vi "gugudan Client.vi"() -> ()   [LabVIEW 2014]
uses:
  <vilib>/Utility/sysdir.llb/System Directory Type.ctl
  <vilib>/FTP/NI_FTP.lvlib
panel:
  out "ip address 3":string=" ip address\r\n   서브넷 마스크 . . . . . . . : 255.255.255.0\r\n   기본 게이트웨이 . . . . . . : 192.168.0.1\r\n\r\n터널 어댑터 isatap.{E2E91750-802C-47E4-94E7-F6C5BD44A78B}:\r\n\r\n   미디어 상태 . . . . . . . . : 미디어 연결 끊김\r\n   연결별 DNS 접미사. . . . : \r\n\r\n터널 어댑터 로컬 영역 연결* 2:\r\n\r\n   연결별 DNS 접미사. . . . : \r\n   IPv6 주소 . . . . . . . . . : 2001:0:682f:9980:3c40:17a9:3f57:fff6\r\n   링크-로컬 IPv6 주소 . . . . : fe80::3c40:17a9:3f57:fff6%12\r\n   기본 게이트웨이 . . . . . . : ::\r\n"
  out "email 2":string
  out "ip address":string=" ip address\r\n   서브넷 마스크 . . . . . . . : 255.255.255.0\r\n   기본 게이트웨이 . . . . . . : 192.168.0.1\r\n\r\n터널 어댑터 isatap.{E2E91750-802C-47E4-94E7-F6C5BD44A78B}:\r\n\r\n   미디어 상태 . . . . . . . . : 미디어 연결 끊김\r\n   연결별 DNS 접미사. . . . : \r\n\r\n터널 어댑터 로컬 영역 연결* 2:\r\n\r\n   연결별 DNS 접미사. . . . : \r\n   IPv6 주소 . . . . . . . . . : 2001:0:682f:9980:3c40:17a9:3f57:fff6\r\n   링크-로컬 IPv6 주소 . . . . : fe80::3c40:17a9:3f57:fff6%12\r\n   기본 게이트웨이 . . . . . . : ::\r\n"
  in  "제한해제":bool
  out "TIME":string="현재날자,시간"
  out "배열":string[][](array[string])
  out "email":string
  out "abs(x)":i32
  out "문자열":string
  out "스페이스바3 2":string
  out "W 2":string
  out "W":string
  out "1":string
  out "2":string
  out "3":string
  out "스페이스바3":string
  out "key의숫자값":i16[](array[numeric])
  # "서비스를 이용해 주셔 감사합니다."
  # "서비스 종료를 위해서는 관리자 암호를 입력 해야 종료가 가능합니다."
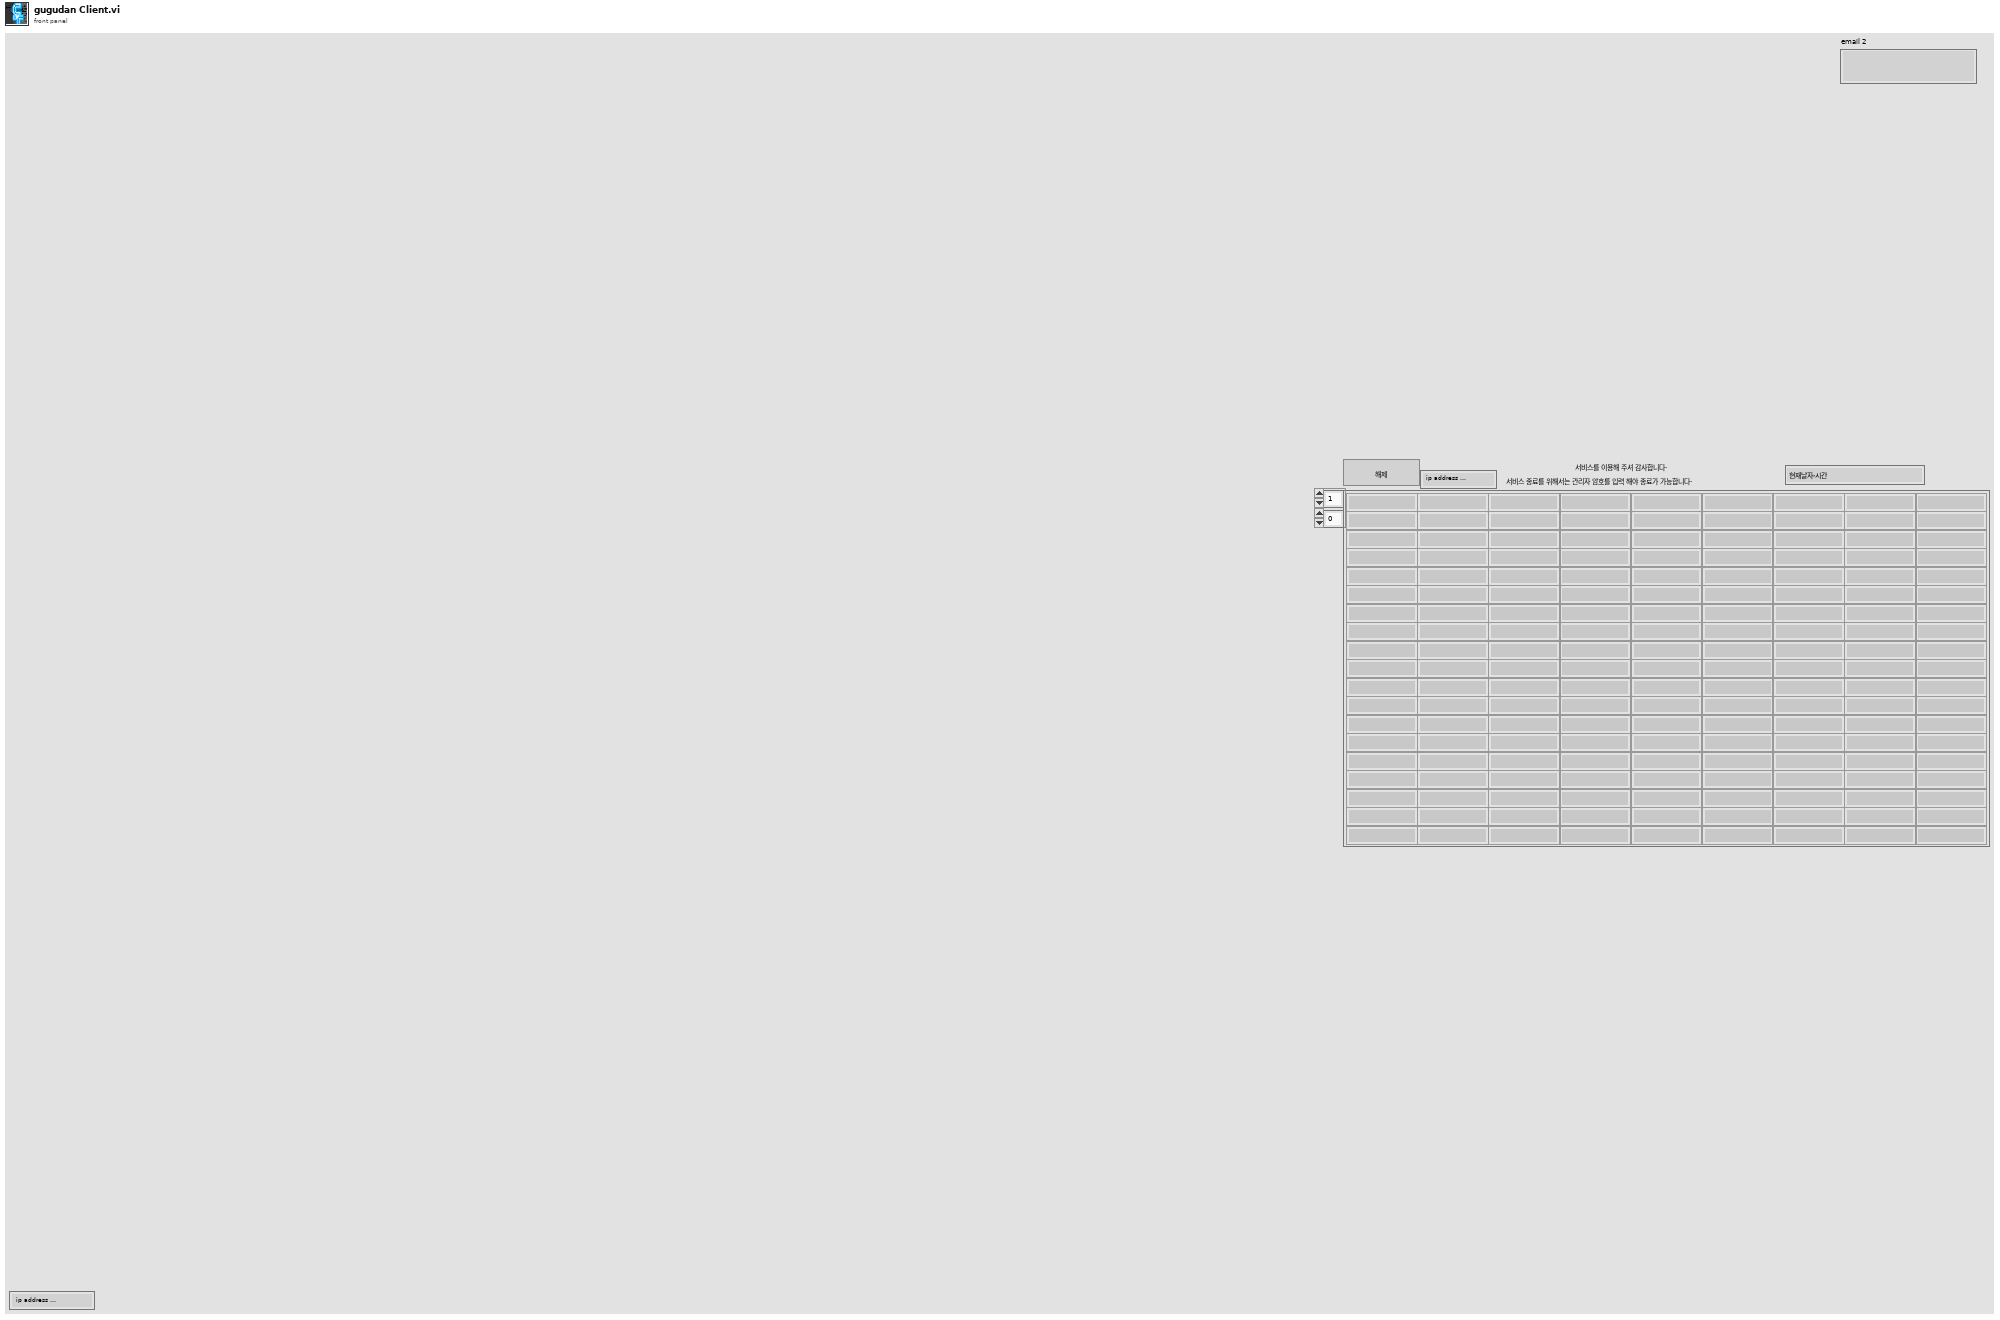
[diagram p1: front panel]
types:
  T1 = enum16{"open", "replace", "create", "open or create", "replace or create", "replace or create with confirmation"}
  T2 = typedef "NI_FTP.lvlib/FTP Session.ctl" = refnum<k5>
  T3 = typedef "System Directory Type.ctl" = i32
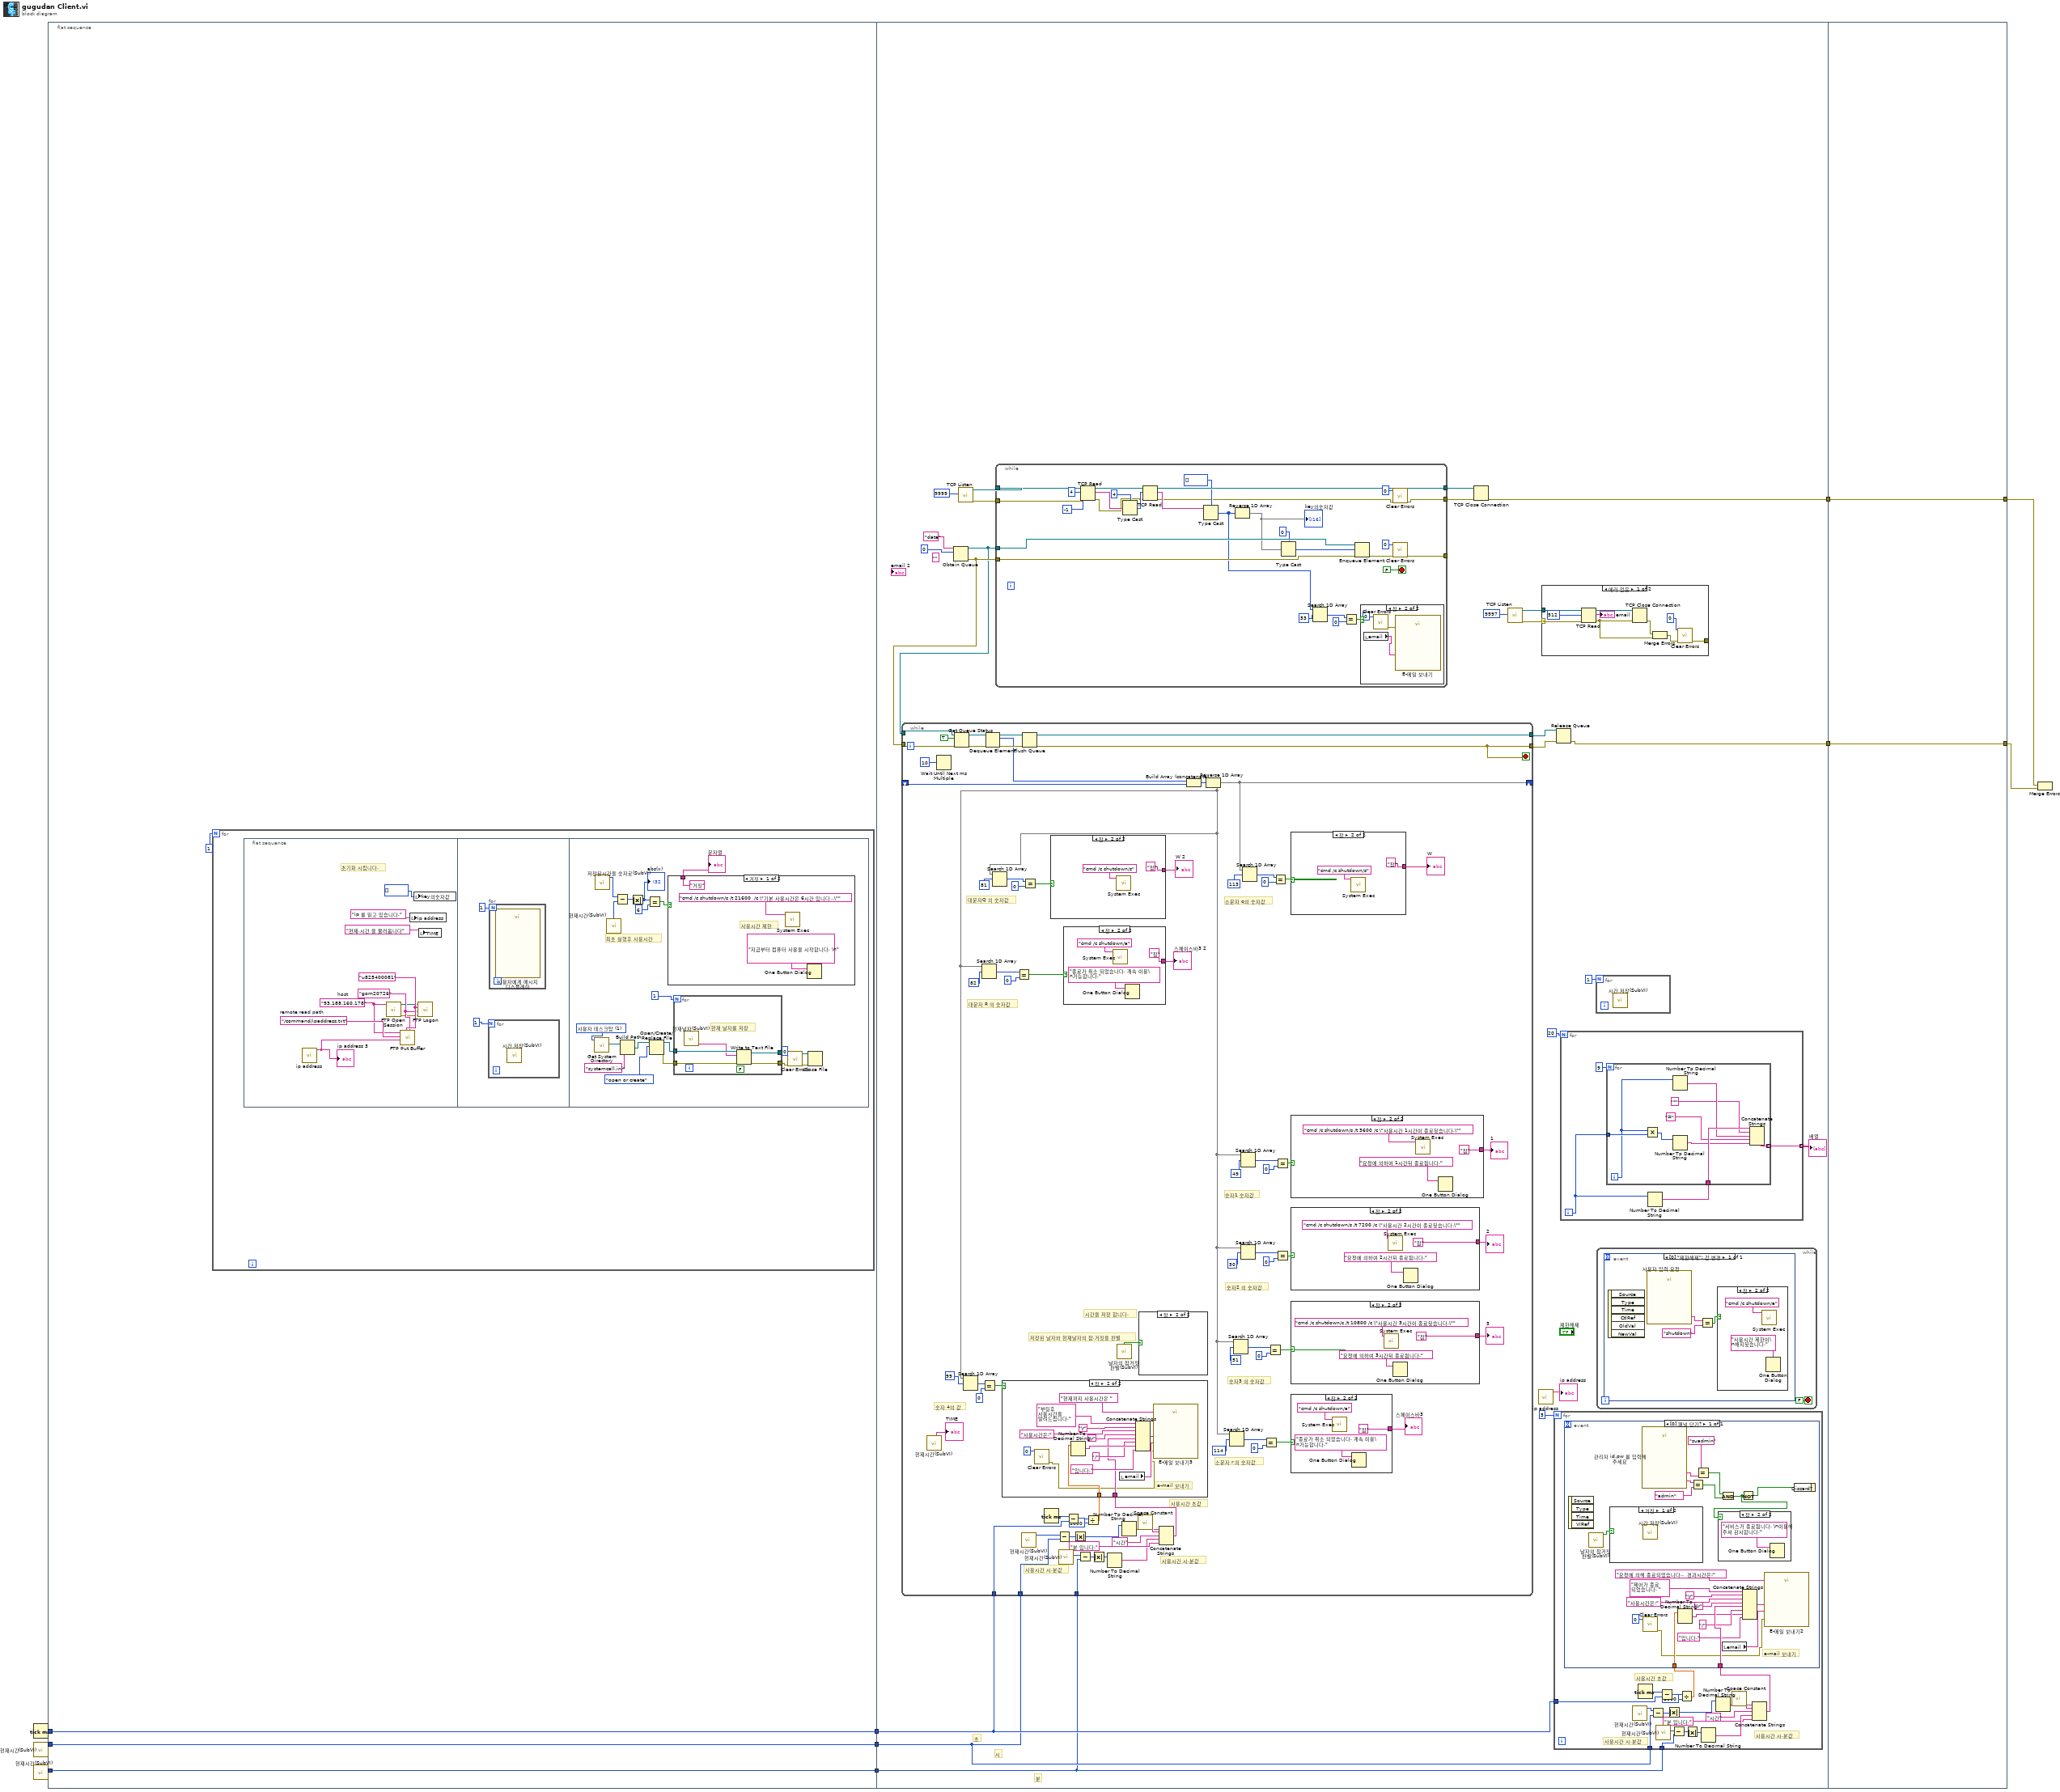
[diagram p0: block diagram]
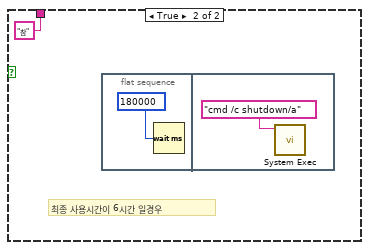
[diagram p2: hidden frame]
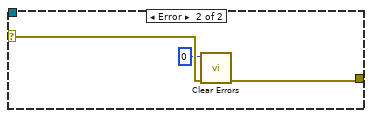
[diagram p4: hidden frame]
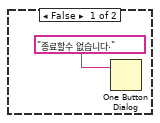
[diagram p6: hidden frame]
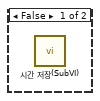
[diagram p8: hidden frame]
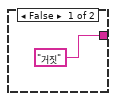
[diagram p9: hidden frame]
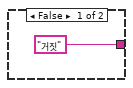
[diagram p10: hidden frame]
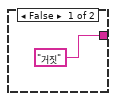
[diagram p11: hidden frame]
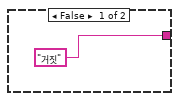
[diagram p12: hidden frame]
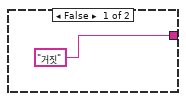
[diagram p13: hidden frame]
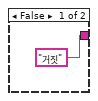
[diagram p14: hidden frame]
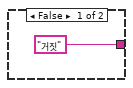
[diagram p15: hidden frame]
diagram:
  n1 = Tick Count (ms)() -> (millisecond timer value=w6:u32)
  n2 = call "현재시간(SubVI).vi"() -> ("시"=w5:i32)  [unwired: 3 in, 8 out]
  n3 = call "현재시간(SubVI).vi"() -> ("분"=w4:i32)  [unwired: 3 in, 8 out]
  n4 = flat-sequence {
    tunnel: [w13] -> w7
    tunnel: w6 -> [w13]
    tunnel: w5 -> [w12]
    tunnel: w4 -> [w11]
    tunnel: [w12] -> w3
    tunnel: [w11] -> w2
    tunnel: [w71] -> w10
    tunnel: [w70] -> w9
    tunnel: w7 -> [w66]
    tunnel: w3 -> [w65]
    tunnel: w2 -> [w64]
    tunnel: w10 -> [w304]
    tunnel: w9 -> [w303]
    tunnel: [w304] -> w8
    tunnel: [w303] -> w1
    frame #0 {
      n5 = for {
        N: 1 -> [_]
        n6 = flat-sequence {
          frame #0 {
            w17 = "gom20726"
            w20 = "u825400081"
            w19 = "/command/ipaddress.txt"  # remote read path
            w18 = "93.188.160.178"  # host
            # "초기화 시킵니다."
            n7 = call "ip address.vi"() -> ("ip address"=w21:string)  [unwired: 11 in]
            "ip address 3" <- w21
            n8 = call <vilib>:"FTP Open Session.vi"("address"=w18) -> ("error out"=w16:errorcluster, "ftp session"=w15:T2)  [unwired: 7 in, 2 out]
            n9 = call <vilib>:"FTP Put Buffer.vi"("password"=w17, "user"=w20, "data"=w21, "remote path"=w19, "host"=w18) -> ()  [unwired: 5 in, 2 out]
            n10 = local write "ip address"("ip 를 읽고 있습니다.") -> ()
            n11 = local write "key의숫자값"(i16[] []) -> ()
            n12 = call <vilib>:"FTP Logon.vi"("error in (no error)"=w16, "password"=w17, "user"=w20, "ftp session"=w15) -> ()  [unwired: 4 in, 4 out]
            n13 = local write "TIME"("현재,시간 을 불러옵니다") -> ()
          }
          frame #1 {
            n14 = for {
              N: 1 -> [_]
              n15 = call "시간 저장(SubVI).vi"() -> ()  [unwired: 12 in]
            }
            n16 = for {
              N: 1 -> [_]
              n17 = call "사용자에게 메시지 디스플레이"() -> ()  [unwired: 10 in, 2 out]
            }
          }
          frame #2 {
            w29 = T3 1 items=["사용자 홈"=0, "사용자 데스크탑"=1, "사용자 문서"=2, "사용자 어플리케이션 데이터"=3, "사용자 환경"=4, "사용자 임시"=5, "퍼블릭 문서"=6, "퍼블릭 어플리케이션 데이터"=7, "퍼블릭 환경"=8, "퍼블릭 캐시"=13, "시스템 코어 라이브러리"=9, "시스템 설치된 라이브러리"=10, "어플리케이션 파일"=11, "부팅 볼륨 루트"=12] ("system directory type")
            # "최초 실행후 사용시간"
            n18 = call <vilib>:"Get System Directory.vi"("system directory type"=w29) -> ("system directory"=w34:path)  [unwired: 10 in]
            n19 = call "저장된시간을 숫자로(SubVI).vi"() -> ("저장된 문자를 숫자로"=w39:i32)  [unwired: 11 in]
            n20 = call "현재시간(SubVI).vi"() -> ("시"=w40:i32)  [unwired: 3 in, 8 out]
            n21 = Subtract(x=w39, y=w40) -> (x-y=w41:i32)
            n22 = Build Path(base path=w34, name or relative path="systemcall.ini" ("이름 또는 상대 경로")) -> (appended path=w32:path)
            n23 = Absolute Value(x=w41) -> (abs(x)=w43:i32)
            "abs(x)" <- w43
            n24 = Equal?(x=w43, y=6) -> (x = y?=w45:bool)
            n25 = Open/Create/Replace File(file path (use dialog)=w32, operation (0:open)=T1."open or create" ("동작(0:open)")) -> (refnum out=w30:refnum<file>, error out=w31:errorcluster)  [unwired: 4 in, 1 out]
            n26 = case shown="거짓" w45 {
              tunnel: ["거짓" "참"] -> w42
              frame False {
                # "사용시간 제한"
                n27 = call <vilib>:"System Exec.vi"("command line"="cmd /c shutdown/s /t 21600  /c \"기본 사용시간은 6시간 입니다..\"" ("standard input")) -> ()  [unwired: 7 in, 4 out]
                n28 = One Button Dialog(message="지금부터 컴퓨터 사용을 시작합니다. \n" ("메시지")) -> ()  [unwired: 1 in, 1 out]
              }
              frame True {
                # "최종 사용시간이 6시간 일경우"
                n29 = flat-sequence {
                  frame #0 {
                    n30 = Wait (ms)(milliseconds to wait=u32 180000 ("대기 시간(ms)")) -> ()  [unwired: 1 out]
                  }
                  frame #1 {
                    n31 = call <vilib>:"System Exec.vi"("command line"="cmd /c shutdown/a" ("standard input")) -> ()  [unwired: 7 in, 4 out]
                  }
                }
              }
            }
            "문자열" <- w42
            n32 = for {
              N: 1 -> [_]
              tunnel: w31 -> [w50]
              tunnel: [w49] -> w36
              tunnel: [w48] -> w35
              tunnel: w30 -> [w47]
              (unwired) FALSE
              # "현재 날자를 저장"
              n33 = call "현재날자(SubVI).vi"() -> ("월,일 을 문자열로"=w46:string)  [unwired: 5 in, 6 out]
              n34 = Write to Text File(file (use dialog)=w47, text=w46, error in=w50) -> (refnum out=w48:refnum<file>, error out=w49:errorcluster)  [unwired: 1 in, 1 out]
            }
            n35 = call <vilib>:"Clear Errors.vi"("error in (no error)"=w36, "specific error code to clear (0: all)"=0) -> ("error out"=w37:errorcluster)  [unwired: 4 in, 1 out]
            n36 = Close File(refnum=w35, error in=w37) -> ()  [unwired: 2 out]
          }
        }
      }
    }
    frame #1 {
      (unwired) ""
      # "초"
      # "분"
      # "시"
      n37 = Obtain Queue(name (unnamed)="data" ("이름(이름없음)"), element data type=i16 0) -> (queue out=w72:refnum<queue>, error out=w73:errorcluster)  [unwired: 3 in, 1 out]
      n38 = while {
        shift-right: [w158] -> _
        shift-left: _ -> [w204]
        tunnel: [w197] -> w75
        tunnel: [w196] -> w74
        tunnel: w72 -> [w203]
        tunnel: w73 -> [w202]
        tunnel: w66 -> [w163]
        tunnel: w65 -> [w162]
        tunnel: w64 -> [w161]
        stop <- w196 stop-if-true
        # "숫자 4의 값"
        # "저장된 날자와 현재날자의 참,거짓을 판별"
        # "시간을 저장 합니다."
        # "사용시간 시,분값"
        # "사용시간 시,분값"
        # "사용시간 초값"
        # "대문자 R 의 숫자값"
        # "대문자Q 의 숫자값"
        # "소문자 r 의 숫자값"
        # "숫자3 의 숫자값"
        # "소문자 q의 숫자값"
        # "숫자1 숫자값"
        # "숫자2 의 숫자값"
        n39 = call "현재시간(SubVI).vi"() -> ("날짜/시간 문자열"=→"TIME":string)  [unwired: 3 in, 8 out]
        n40 = Wait Until Next ms Multiple(millisecond multiple=u32 10) -> ()  [unwired: 1 out]
        n41 = Get Queue Status(queue=w203, return elements? (F)=TRUE ("원소 반환? (거짓)"), error in (no error)=w202) -> (queue out=w201:refnum<queue>, error out=w200:errorcluster)  [unwired: 6 out]
        n42 = Dequeue Element(queue=w201, error in (no error)=w200) -> (queue out=w198:refnum<queue>, element=w195:i16, error out=w199:errorcluster)  [unwired: 1 in, 1 out]
        n43 = call "현재시간(SubVI).vi"() -> ("시"=w165:i32)  [unwired: 3 in, 8 out]
        n44 = Flush Queue(queue=w198, error in (no error)=w199) -> (queue out=w197:refnum<queue>, error out=w196:errorcluster)  [unwired: 1 out]
        n45 = Tick Count (ms)() -> (millisecond timer value=w164:u32)
        n46 = Subtract(x=w165, y=w162) -> (x-y=w167:i32)
        n47 = call "현재시간(SubVI).vi"() -> ("분"=w166:i32)  [unwired: 3 in, 8 out]
        n48 = Subtract(x=w164, y=w163) -> (x-y=w176:u32)
        n49 = Absolute Value(x=w167) -> (abs(x)=w169:i32)
        n50 = Subtract(x=w166, y=w161) -> (x-y=w168:i32)
        n51 = Divide(x=w176, y=u32 1000) -> (x/y=w160:dbl)
        n52 = Absolute Value(x=w168) -> (abs(x)=w170:i32)
        n53 = Number To Decimal String(number=w170) -> (decimal integer string=w172:string)  [unwired: 1 in]
        n54 = call "날자의 참거짓 판별(SubVI).vi"() -> ("불리언"=w182:bool)  [unwired: 9 in, 2 out]
        n55 = Number To Decimal String(number=w169) -> (decimal integer string=w174:string)  [unwired: 1 in]
        n56 = call <vilib>:"Space Constant.vi"() -> ("String"=w175:string)
        n57 = case shown="참" w182 {
          frame False {
            n58 = call "시간 저장(SubVI).vi"() -> ()  [unwired: 12 in]
          }
          frame True {
          }
        }
        n59 = Concatenate Strings(w174, w175, "시간", w172, "분 입니다.") -> (w159:string)
        n60 = Build Array (concatenate)(w195, w204) -> (w193:i16[])
        n61 = Reverse 1D Array(array=w193) -> (reversed array=w158:i16[])
        n62 = Search 1D Array(1D array=w158, element=i16 99 ("원소")) -> (index of element=w180:i32)  [unwired: 1 in]
        n63 = Search 1D Array(1D array=w158, element=i16 82 ("원소")) -> (index of element=w185:i32)  [unwired: 1 in]
        n64 = Equal?(x=w180, y=0) -> (x = y?=w178:bool)
        n65 = Search 1D Array(1D array=w158, element=i16 81 ("원소")) -> (index of element=w190:i32)  [unwired: 1 in]
        n66 = case shown="참" w178 {
          tunnel: w160 -> [_ w235]
          tunnel: w159 -> [_ w234]
          frame False {
          }
          frame True {
            # "e-mail 보내기"
            n67 = call <vilib>:"Clear Errors.vi"("specific error code to clear (0: all)"=0) -> ("error out"=w231:errorcluster)  [unwired: 5 in, 1 out]
            n68 = Number To Decimal String(number=w235) -> (decimal integer string=w243:string)  [unwired: 1 in]
            n69 = local read "email"() -> (w233:string)
            n70 = Concatenate Strings("부팅후 사용시간을 알려드립니다." ("문자열"), "\r", "사용시간은:", "\r", w234, "/", w243, "입니다.") -> (w240:string)
            n71 = call "E-메일 보내기3"("error in"=w231, "Message"=w240, "Subject"="현재까지 사용시간은 ", "Recipients"=w233) -> ()  [unwired: 7 in, 1 out]
          }
        }
        n72 = Equal?(x=w185, y=0) -> (x = y?=w187:bool)
        n73 = Equal?(x=w190, y=0) -> (x = y?=w188:bool)
        n74 = case shown="참" w188 {
          tunnel: ["거짓" "참"] -> w192
          frame False {
          }
          frame True {
            n75 = call <vilib>:"System Exec.vi"("command line"="cmd /c shutdown/s" ("standard input")) -> ()  [unwired: 7 in, 4 out]
          }
        }
        "W 2" <- w192
        n76 = case shown="참" w187 {
          tunnel: ["거짓" "참"] -> w183
          frame False {
          }
          frame True {
            n77 = call <vilib>:"System Exec.vi"("command line"="cmd /c shutdown/a" ("standard input")) -> ()  [unwired: 7 in, 4 out]
            n78 = One Button Dialog(message="종료가 취소 되었습니다. 계속 이용\n가능합니다." ("메시지")) -> ()  [unwired: 1 in, 1 out]
          }
        }
        "스페이스바3 2" <- w183
        n79 = Search 1D Array(1D array=w158, element=i16 114 ("원소")) -> (index of element=w209:i32)  [unwired: 1 in]
        n80 = Search 1D Array(1D array=w158, element=i16 51 ("원소")) -> (index of element=w214:i32)  [unwired: 1 in]
        n81 = Search 1D Array(1D array=w158, element=i16 49 ("원소")) -> (index of element=w225:i32)  [unwired: 1 in]
        n82 = Search 1D Array(1D array=w158, element=i16 50 ("원소")) -> (index of element=w218:i32)  [unwired: 1 in]
        n83 = Search 1D Array(1D array=w158, element=i16 113 ("원소")) -> (index of element=w228:i32)  [unwired: 1 in]
        n84 = Equal?(x=w209, y=0) -> (x = y?=w211:bool)
        n85 = Equal?(x=w214, y=0) -> (x = y?=w212:bool)
        n86 = Equal?(x=w228, y=0) -> (x = y?=w226:bool)
        n87 = Equal?(x=w225, y=0) -> (x = y?=w223:bool)
        n88 = Equal?(x=w218, y=0) -> (x = y?=w220:bool)
        n89 = case shown="참" w226 {
          tunnel: ["거짓" "참"] -> w230
          frame False {
          }
          frame True {
            n90 = call <vilib>:"System Exec.vi"("command line"="cmd /c shutdown/s" ("standard input")) -> ()  [unwired: 7 in, 4 out]
          }
        }
        "W" <- w230
        n91 = case shown="참" w223 {
          tunnel: ["거짓" "참"] -> w224
          frame False {
          }
          frame True {
            n92 = call <vilib>:"System Exec.vi"("command line"="cmd /c shutdown/s /t 3600 /c \"사용시간 1시간이 종료됫습니다.\"" ("standard input")) -> ()  [unwired: 7 in, 4 out]
            n93 = One Button Dialog(message="요청에 의하여 1시간뒤 종료됩니다." ("메시지")) -> ()  [unwired: 1 in, 1 out]
          }
        }
        "1" <- w224
        n94 = case shown="참" w220 {
          tunnel: ["거짓" "참"] -> w219
          frame False {
          }
          frame True {
            n95 = call <vilib>:"System Exec.vi"("command line"="cmd /c shutdown/s /t 7200 /c \"사용시간 2시간이 종료됫습니다.\"" ("standard input")) -> ()  [unwired: 7 in, 4 out]
            n96 = One Button Dialog(message="요청에 의하여 2시간뒤 종료됩니다." ("메시지")) -> ()  [unwired: 1 in, 1 out]
          }
        }
        "2" <- w219
        n97 = case shown="참" w212 {
          tunnel: ["거짓" "참"] -> w194
          frame False {
          }
          frame True {
            n98 = call <vilib>:"System Exec.vi"("command line"="cmd /c shutdown/s /t 10800 /c \"사용시간 3시간이 종료됫습니다.\"" ("standard input")) -> ()  [unwired: 7 in, 4 out]
            n99 = One Button Dialog(message="요청에 의하여 3시간뒤 종료됩니다." ("메시지")) -> ()  [unwired: 1 in, 1 out]
          }
        }
        "3" <- w194
        n100 = case shown="참" w211 {
          tunnel: ["거짓" "참"] -> w207
          frame False {
          }
          frame True {
            n101 = call <vilib>:"System Exec.vi"("command line"="cmd /c shutdown/a" ("standard input")) -> ()  [unwired: 7 in, 4 out]
            n102 = One Button Dialog(message="종료가 취소 되었습니다. 계속 이용\n가능합니다." ("메시지")) -> ()  [unwired: 1 in, 1 out]
          }
        }
        "스페이스바3" <- w207
      }
      n103 = call <vilib>:"TCP Listen.vi"("port"=u16 9999) -> ("error out"=w68:errorcluster, "connection ID"=w78:refnum<k5>)  [unwired: 6 in, 3 out]
      n104 = while {
        tunnel: w78 -> [w271]
        tunnel: [w299] -> w79
        tunnel: w72 -> [w292]
        tunnel: w73 -> [w291]
        tunnel: [w277] -> w69
        tunnel: w68 -> [w283]
        tunnel: [w274] -> _
        stop <- FALSE stop-if-true
        n105 = TCP Read(connection ID=w271, bytes to read=4, error in (no error)=w283, 9:-1 ("타임아웃 ms (25000)")) -> (connection ID out=w295:refnum<k5>, data out=w297:string, error out=w284:errorcluster)  [unwired: 1 in]
        n106 = Type Cast(type=4 ("bytes to read"), x=w297) -> (*(type *) &x=w289:i32)
        n107 = TCP Read(connection ID=w295, bytes to read=w289, error in (no error)=w284) -> (connection ID out=w299:refnum<k5>, data out=w290:string, error out=w276:errorcluster)  [unwired: 2 in]
        n108 = Type Cast(type=i16[] [], x=w290) -> (*(type *) &x=w279:i16[])
        n109 = Reverse 1D Array(array=w279) -> (reversed array=w285:i16[])
        "key의숫자값" <- w285
        n110 = Type Cast(type=i16 0, x=w285) -> (*(type *) &x=w287:i16)
        n111 = Search 1D Array(1D array=w279, element=i16 53 ("원소")) -> (index of element=w282:i32)  [unwired: 1 in]
        n112 = Equal?(x=w282, y=0) -> (x = y?=w278:bool)
        n113 = Enqueue Element(queue=w292, element=w287, error in (no error)=w291) -> (error out=w275:errorcluster)  [unwired: 1 in, 2 out]
        n114 = case shown="참" w278 {
          frame False {
          }
          frame True {
            n115 = local read "email"() -> (w302:string)
            n116 = call <vilib>:"Clear Errors.vi"("specific error code to clear (0: all)"=0) -> ("error out"=w300:errorcluster)  [unwired: 5 in, 1 out]
            n117 = call "E-메일 보내기"("error in"=w300, "Recipients"=w302) -> ()  [unwired: 9 in, 1 out]
          }
        }
        n118 = call <vilib>:"Clear Errors.vi"("error in (no error)"=w276, "specific error code to clear (0: all)"=0) -> ("error out"=w277:errorcluster)  [unwired: 4 in, 1 out]
        n119 = call <vilib>:"Clear Errors.vi"("error in (no error)"=w275, "specific error code to clear (0: all)"=0) -> ("error out"=w274:errorcluster)  [unwired: 4 in, 1 out]
      }
      n120 = TCP Close Connection(connection ID=w79, error in (no error)=w69) -> (error out=w70:errorcluster)  [unwired: 1 in, 1 out]
      n121 = call <vilib>:"TCP Listen.vi"("port"=u16 9997) -> ("error out"=w61:errorcluster, "connection ID"=w62:refnum<k5>)  [unwired: 6 in, 3 out]
      n122 = call "ip address.vi"() -> ("ip address"=→"ip address":string)  [unwired: 11 in]
      n123 = case shown="에러 없음" w61 {
        selector: w61 -> [w105 w111]
        tunnel: [w102 w112] -> _
        tunnel: w62 -> [w109 _]
        frame No Error {
          n124 = TCP Read(connection ID=w109, bytes to read=512, error in (no error)=w105) -> (connection ID out=w104:refnum<k5>, data out=→"email":string, error out=w103:errorcluster)  [unwired: 2 out]
          n125 = TCP Close Connection(connection ID=w104, error in (no error)=w103) -> (error out=w106:errorcluster)  [unwired: 2 out]
          n126 = Merge Errors(w106, w103) -> (w101:errorcluster)
          n127 = call <vilib>:"Clear Errors.vi"("error in (no error)"=w101, "specific error code to clear (0: all)"=0) -> ("error out"=w102:errorcluster)  [unwired: 4 in, 1 out]
        }
        frame Error {
          n128 = call <vilib>:"Clear Errors.vi"("error in (no error)"=w111, "specific error code to clear (0: all)"=0) -> ("error out"=w112:errorcluster)  [unwired: 4 in, 1 out]
        }
      }
      n129 = for {
        N: 5 -> [_]
        tunnel: w66 -> [w130]
        tunnel: w65 -> [w128]
        tunnel: w64 -> [w126]
        # "사용시간 시,분값"
        # "사용시간 시,분값"
        # "사용시간 초값"
        n130 = call "현재시간(SubVI).vi"() -> ("시"=w129:i32)  [unwired: 3 in, 8 out]
        n131 = Tick Count (ms)() -> (millisecond timer value=w131:u32)
        n132 = Subtract(x=w129, y=w128) -> (x-y=w125:i32)
        n133 = call "현재시간(SubVI).vi"() -> ("분"=w127:i32)  [unwired: 3 in, 8 out]
        n134 = Subtract(x=w131, y=w130) -> (x-y=w116:u32)
        n135 = Absolute Value(x=w125) -> (abs(x)=w123:i32)
        n136 = Subtract(x=w127, y=w126) -> (x-y=w124:i32)
        n137 = Divide(x=w116, y=u32 1000) -> (x/y=w114:dbl)
        n138 = Absolute Value(x=w124) -> (abs(x)=w122:i32)
        n139 = Number To Decimal String(number=w122) -> (decimal integer string=w120:string)  [unwired: 1 in]
        n140 = Number To Decimal String(number=w123) -> (decimal integer string=w118:string)  [unwired: 1 in]
        n141 = call <vilib>:"Space Constant.vi"() -> ("String"=w117:string)
        n142 = Concatenate Strings(w118, w117, "시간", w120, "분 입니다.") -> (w113:string)
        n143 = event shown="[0] 패널 닫기?" {
          selector: _ -> [_]
          dyn-events: _ -> [_]
          timeout: _ -> [_]
          tunnel: w114 -> [w146]
          tunnel: w113 -> [w139]
          event Panel Close? {
            # "e-mail 보내기"
            n144 = event-data() -> ()  [unwired: 1 in, 4 out]
            n145 = call "날자의 참거짓 판별(SubVI).vi"() -> ("불리언"=w135:bool)  [unwired: 9 in, 2 out]
            n146 = case shown="거짓" w135 {
              frame False {
                n147 = call "시간 저장(SubVI).vi"() -> ()  [unwired: 12 in]
              }
              frame True {
              }
            }
            n148 = call "관리자 id.pw 를 입력해 주세요"() -> ("PW"=w154:string, "ID"=w151:string)  [unwired: 16 in, 2 out]
            n149 = call <vilib>:"Clear Errors.vi"("specific error code to clear (0: all)"=0) -> ("error out"=w133:errorcluster)  [unwired: 5 in, 1 out]
            n150 = Number To Decimal String(number=w146) -> (decimal integer string=w137:string)  [unwired: 1 in]
            n151 = Equal?(x=w154, y="admin") -> (x = y?=w150:bool)
            n152 = Equal?(x="suadmin", y=w151) -> (x = y?=w149:bool)
            n153 = And(x=w149, y=w150) -> (x .and. y?=w147:bool)
            n154 = case shown="참" w147 {
              frame False {
                n155 = One Button Dialog(message="종료할수 없습니다." ("메시지")) -> ()  [unwired: 1 in, 1 out]
              }
              frame True {
                n156 = One Button Dialog(message="서비스가 종료됩니다. \n이용해 주셔 감사합니다." ("메시지")) -> ()  [unwired: 1 in, 1 out]
              }
            }
            n157 = local read "email"() -> (w134:string)
            n158 = Not(x=w147) -> (.not. x?=w148:bool)
            n159 = Concatenate Strings("제어가 종료 되었습니다. " ("문자열"), "\r", "사용시간은:", "\r", w139, "/", w137, "입니다.") -> (w141:string)
            n160 = call "E-메일 보내기2"("error in"=w133, "Message"=w141, "Subject"="요청에 의해 종료되었습니다,.  경과시간은:", "Recipients"=w134) -> ()  [unwired: 7 in, 1 out]
            n161 = event-data("Discard?"=w148) -> ()  [unwired: 1 in, 1 out]
          }
        }
      }
      n162 = Release Queue(queue=w75, error in (no error)=w74) -> (error out=w71:errorcluster)  [unwired: 1 in, 2 out]
      n163 = for {
        N: 20 -> [_]
        tunnel: [w87] -> w59 mode=indexing
        i -> [w89]
        n164 = Number To Decimal String(number=w89) -> (decimal integer string=w88:string)  [unwired: 1 in]
        n165 = for {
          N: 9 -> [_]
          tunnel: w89 -> [w99]
          tunnel: w88 -> [w97]
          tunnel: [w92] -> w87 mode=indexing
          i -> [w91]
          n166 = Multiply(x=w91, y=w99) -> (x*y=w98:i32)
          n167 = Number To Decimal String(number=w91) -> (decimal integer string=w96:string)  [unwired: 1 in]
          n168 = Number To Decimal String(number=w98) -> (decimal integer string=w93:string)  [unwired: 1 in]
          n169 = Concatenate Strings(w97, "*", w96, "=", w93) -> (w92:string)
        }
      }
      "배열" <- w59
      n170 = for {
        N: 1 -> [_]
        n171 = call "시간 저장(SubVI).vi"() -> ()  [unwired: 12 in]
      }
      n172 = while {
        stop <- FALSE stop-if-true
        n173 = event shown="[0] \"제한해제\": 값 변경" {
          selector: _ -> [_]
          dyn-events: _ -> [_]
          timeout: _ -> [_]
          event "제한해제": Value Change {
            n174 = event-data() -> ()  [unwired: 1 in, 6 out]
            n175 = call "사용자 입력 요청"() -> ("종료 취소"=w83:string)  [unwired: 17 in, 2 out]
            n176 = Equal?(x=w83, y="shutdown") -> (x = y?=w82:bool)
            n177 = case shown="참" w82 {
              frame False {
              }
              frame True {
                n178 = call <vilib>:"System Exec.vi"("command line"="cmd /c shutdown/a" ("standard input")) -> ()  [unwired: 7 in, 4 out]
                n179 = One Button Dialog(message="사용시간 제한이\n해지됫습니다." ("메시지")) -> ()  [unwired: 1 in, 1 out]
              }
            }
          }
        }
      }
    }
    frame #2 {
    }
  }
  n180 = Merge Errors(w1, w8) -> ()  [unwired: 1 out]
